vi "HeidenhainParamsGet_FGV.vi"(8 "error in":errorcluster, 10 "FGV_Control":enum16{"Set", "Get"}(ring), 11 "in":T1) -> (0 "error out":errorcluster, 3 "out":T1)   [LabVIEW 2011]
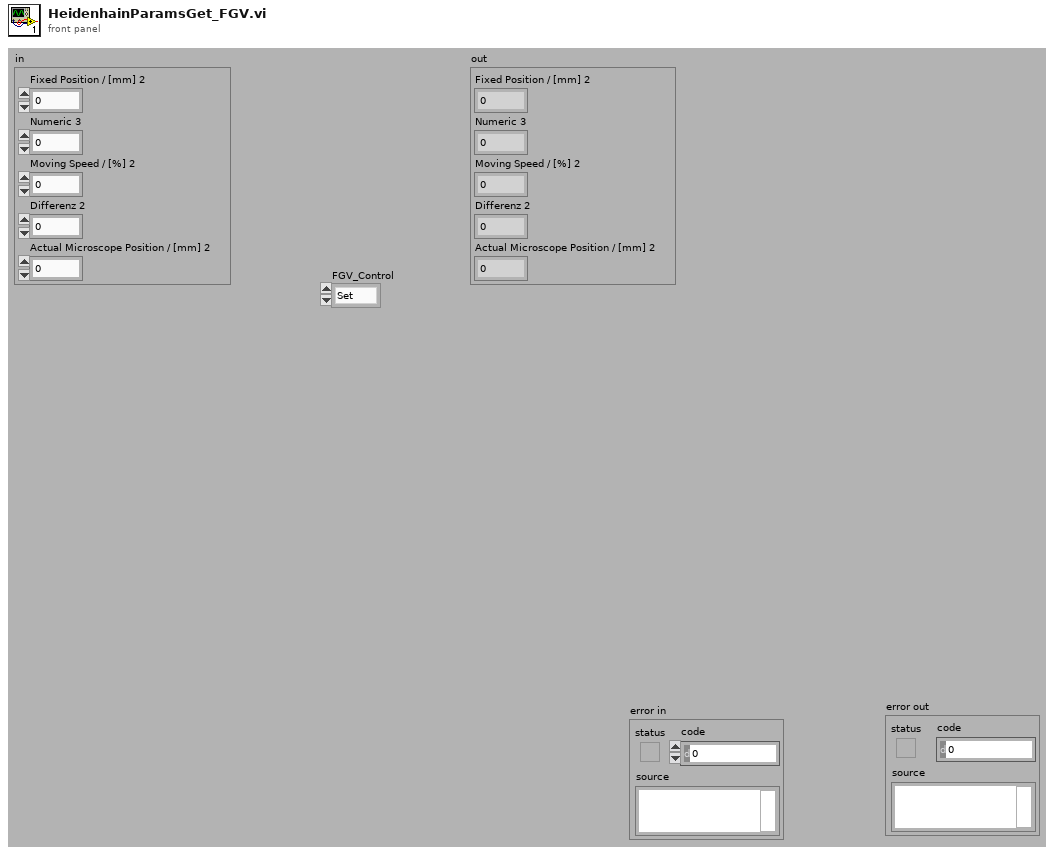
[diagram p1: front panel]
types:
  T1 = cluster{"Fixed Position / [mm] 2":dbl, "Numeric 3":dbl, "Moving Speed / [%] 2":i8, "Differenz 2":dbl, "Actual Microscope Position / [mm] 2":dbl}
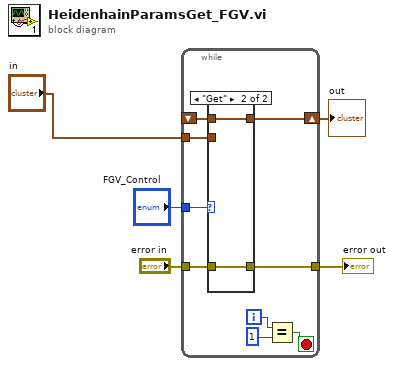
[diagram p0: block diagram]
diagram:
  n1 = while {
    tunnel: "in" -> [w14]
    shift-right: [w13] -> w1
    shift-left: _ -> [w12]
    tunnel: "error in" -> [w8]
    tunnel: [w7] -> w4
    tunnel: "FGV_Control" -> [w6]
    i -> [w9]
    stop <- w10 stop-if-true
    n2 = case shown="\"Get\"" w6 {
      tunnel: w14 -> [w16 _]
      tunnel: [w16 w18] -> w13
      tunnel: w12 -> [_ w18]
      tunnel: w8 -> [w15 w17]
      tunnel: [w15 w17] -> w7
      frame "Set", Default {
      }
      frame "Get" {
      }
    }
    n3 = Equal?(x=w9, y=1) -> (x = y?=w10:bool)
  }
  "error out" <- w4
  "out" <- w1
